vi "LED design.vi"() -> ()   [LabVIEW 2015]
panel:
  in  "Tab Control":enum32{"Page 1", "Page 2"}(tab)
  in  "auto pattern":bool=TRUE
  out "green pattern":u64 format="%016x"
  in  "Array 3":bool[][](array[boolean])
  in  "stop":bool
  out "Array 4":bool[][](array[boolean])
  in  "pattern loop time [ms] 2":u32(slide)=500 scale=10.0..1000.0
  out "Array":bool[][](array[boolean])
  in  "ESC 2":bool
  in  "pattern loop time [ms]":u32(slide)=500 scale=10.0..1000.0
  in  "ESC":bool
  # "Pardeep Kumar"
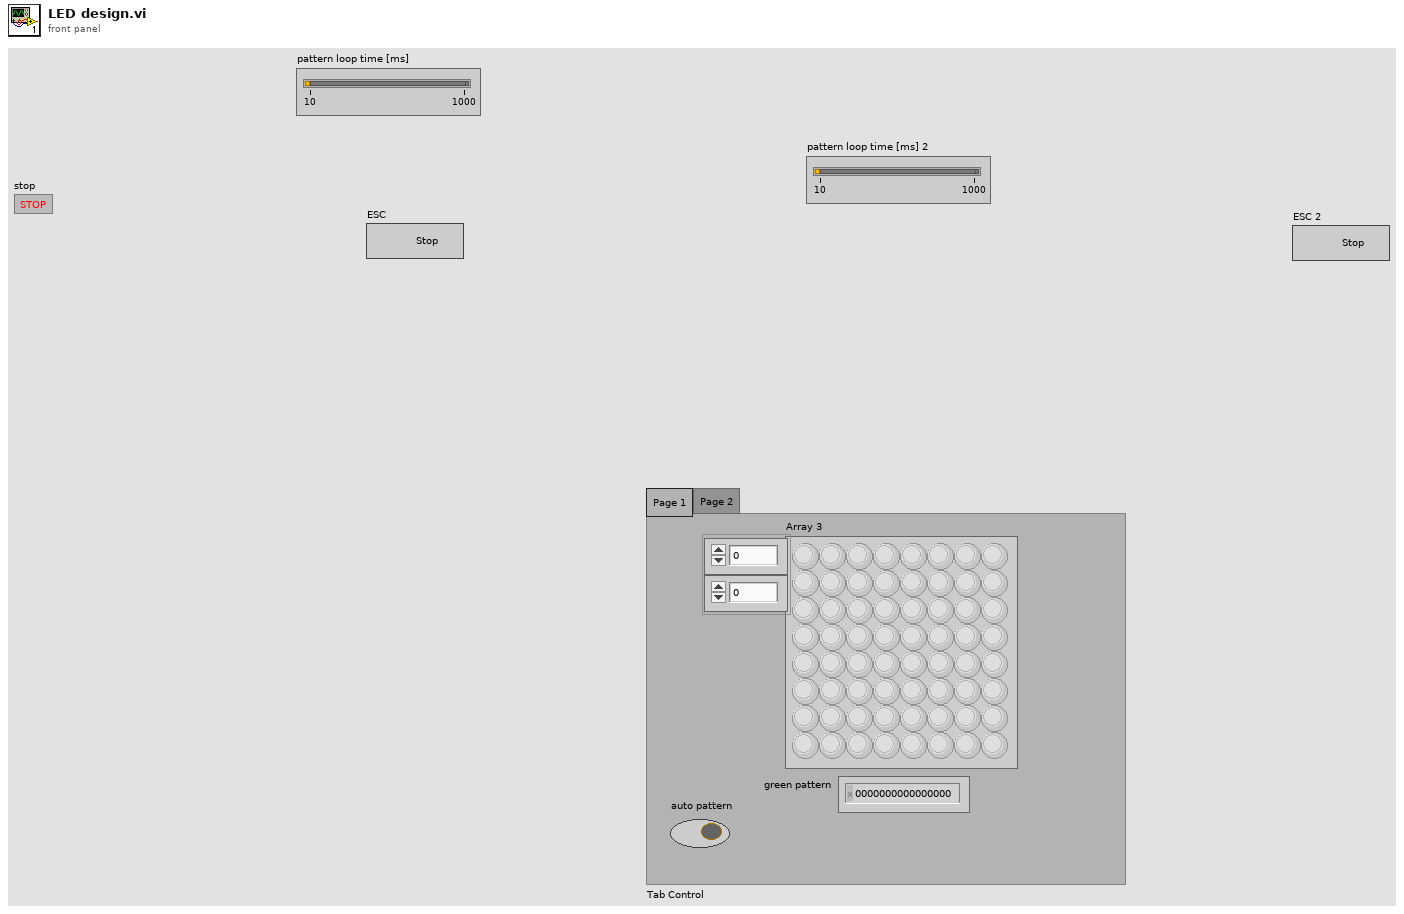
[diagram p1: front panel]
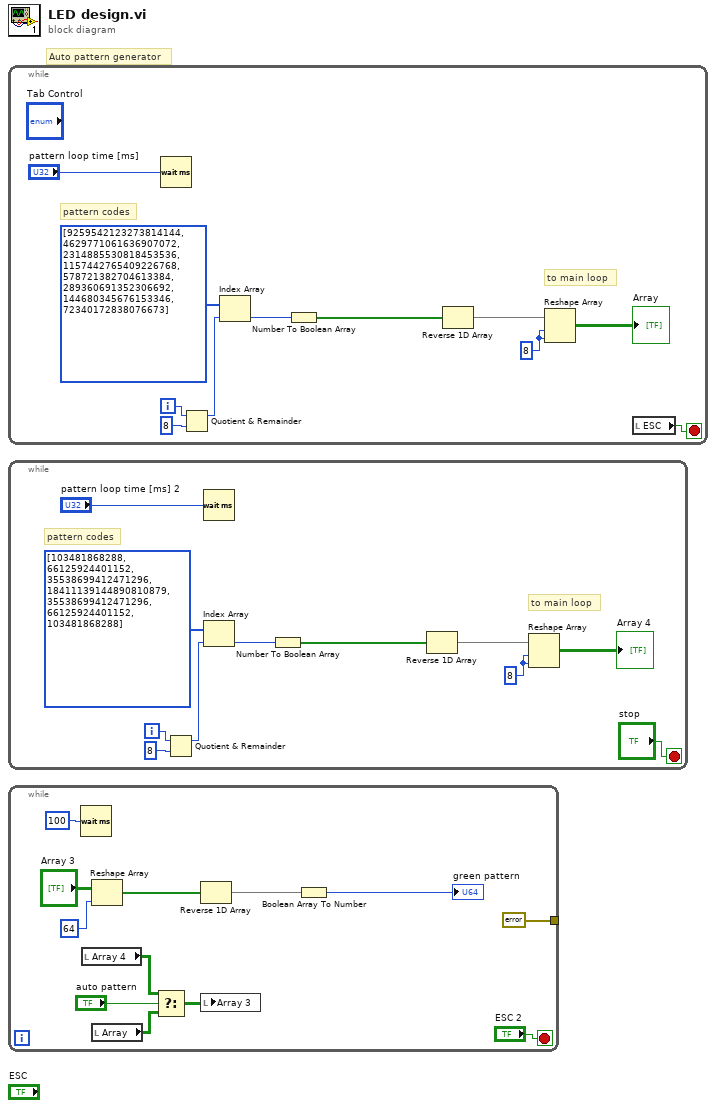
[diagram p0: block diagram]
diagram:
  # "Auto pattern generator"
  n1 = while {
    i -> [w1]
    stop <- w4 stop-if-true
    w10 = 8 ("dimension size")
    # "to main loop"
    # "pattern codes"
    n2 = Wait (ms)(milliseconds to wait="pattern loop time [ms]") -> ()  [unwired: 1 out]
    n3 = Quotient & Remainder(x=w1, y=8) -> (x-y*floor(x/y)=w6:i32)  [unwired: 1 out]
    n4 = Index Array "Index Array"(array=u64[] [9259542123273814144, 4629771061636907072, 2314885530818453536, 1157442765409226768, 578721382704613384, 289360691352306692, 144680345676153346, 72340172838076673], index=w6) -> (element=w7:u64)
    n5 = Number To Boolean Array(number=w7) -> (Boolean array=w8:bool[])
    n6 = Reverse 1D Array(array=w8) -> (reversed array=w9:bool[])
    n7 = Reshape Array "Reshape Array"(w9, w10, w10) -> (→"Array":bool[][])
    n8 = local read "ESC"() -> (w4:bool)
  }
  n9 = while {
    i -> [w13]
    stop <- "stop" stop-if-true
    w21 = 8 ("dimension size")
    # "to main loop"
    # "pattern codes"
    n10 = Quotient & Remainder(x=w13, y=8) -> (x-y*floor(x/y)=w17:i32)  [unwired: 1 out]
    n11 = Wait (ms)(milliseconds to wait="pattern loop time [ms] 2") -> ()  [unwired: 1 out]
    n12 = Index Array "Index Array"(array=u64[] [103481868288, 66125924401152, 35538699412471296, 18411139144890810879, 35538699412471296, 66125924401152, 103481868288], index=w17) -> (element=w18:u64)
    n13 = Number To Boolean Array(number=w18) -> (Boolean array=w19:bool[])
    n14 = Reverse 1D Array(array=w19) -> (reversed array=w20:bool[])
    n15 = Reshape Array "Reshape Array"(w20, w21, w21) -> (→"Array 4":bool[][])
  }
  n16 = while {
    tunnel: [errorcluster {"status"=FALSE, "code"=0, "source"=""} ("error constant")] -> _
    stop <- "ESC 2" stop-if-true
    n17 = Wait (ms)(milliseconds to wait=u32 100) -> ()  [unwired: 1 out]
    n18 = local read "Array 4"() -> (w25:bool[][])
    n19 = Reshape Array "Reshape Array"("Array 3", 64 ("dimension size")) -> (w32:bool[])
    n20 = local read "Array"() -> (w23:bool[][])
    n21 = Select(t=w25, s="auto pattern", f=w23) -> (s? t:f=w24:bool[][])
    n22 = Reverse 1D Array(array=w32) -> (reversed array=w33:bool[])
    n23 = local write "Array 3"(w24) -> ()
    n24 = Boolean Array To Number(Boolean array=w33) -> (number=→"green pattern":u64)
  }
